vi "Floor_Negative16.vi"(10 "Baseline U16":u16, 11 "Input Value":u16) -> (3 "Output Value":u16)   [LabVIEW 2012]
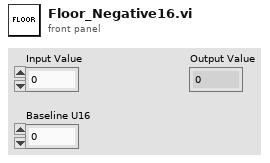
[diagram p1: front panel]
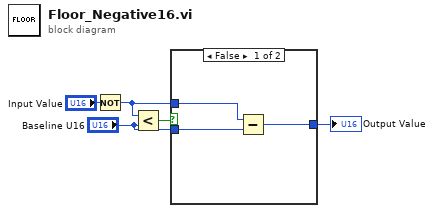
[diagram p0: block diagram]
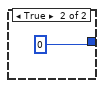
[diagram p2: hidden frame]
diagram:
  n1 = Not(x="Input Value") -> (.not. x?=w3:u16)
  n2 = Less?(x=w3, y="Baseline U16") -> (x < y?=w4:bool)
  n3 = case shown="False" w4 {
    tunnel: w3 -> [w8 _]
    tunnel: "Baseline U16" -> [w7 _]
    tunnel: [w6 i16 0] -> w1
    frame False {
      n4 = Subtract(x=w8, y=w7) -> (x-y=w6:u16)
    }
    frame True {
    }
  }
  "Output Value" <- w1
